vi "Move to Wavelength Inner (TRIAX).vi"(7 "Mono System # (0)":T1, 8 "error in (no error)":errorcluster, 10 "wavelength":dbl[unit], 11 "VISA resource name":refnum<visa-resource-name>) -> (0 "error out":errorcluster, 3 "VISA resource name out":refnum<visa-resource-name>)   [LabVIEW 2012, in "JY-SPEX-TRIAX.lvlib"]
doc: "Moves the spectrometer's grating to a specific wavelength according to the base grating (1200 grooves/mm).\n\n<B>Note: only works with TRIAX series monochromators.</B>"
uses:
  JY-SPEX-TRIAX.lvlib
  controls.llb/Monochromator System Number.ctl
  Spectrometer Config.vi
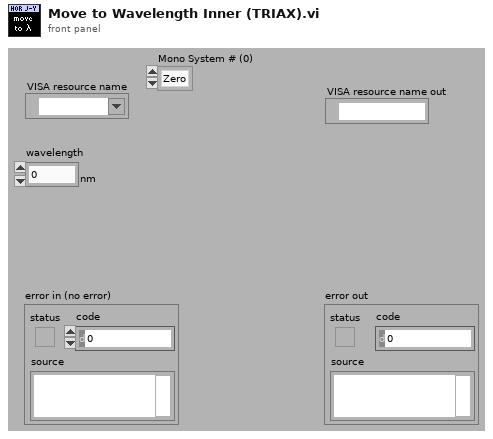
[diagram p1: front panel]
types:
  T1 = typedef "JY-SPEX-TRIAX.lvlib/Monochromator System Number.ctl" = enum16{"Zero", "One"}
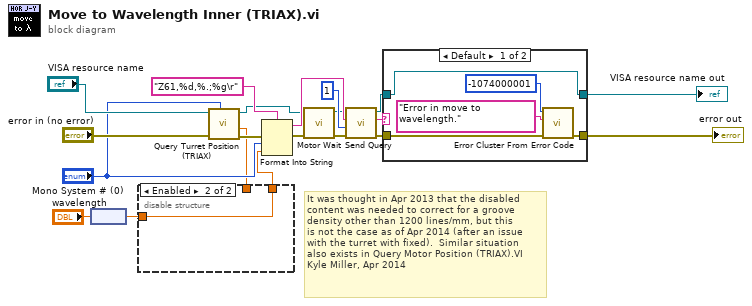
[diagram p0: block diagram]
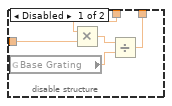
[diagram p2: hidden frame]
diagram:
  # "It was thought in Apr 2013 that the disabled\ncontent was needed to correct for a groove\ndensity other than 1200 lines/mm, but this\nis not the case as of Apr 2014 (after an issue\nwith the turret with fixed).  Similar situation\nalso exists in Query Motor Position (TRIAX).VI\nKyle Miller, Apr 2014"
  n1 = node("wavelength") -> (w3:dbl)
  n2 = call "Query Turret Position (TRIAX).vi"("Mono System # (0)"="Mono System # (0)", "error in (no error)"="error in (no error)", "VISA resource name"="VISA resource name") -> ("error out"=w7:errorcluster, "Groove Density"=w2:dbl[unit], "VISA resource name out"=w4:refnum<visa-resource-name>)  [unwired: 4 in, 2 out]
  n3 = disable-structure shown="Enabled" {
    disable-tunnel: w3 -> [w25 w26]
    disable-tunnel: w2 -> [w24 _]
    disable-tunnel: [w21 w26] -> w1
    frame Disabled {
      n4 = global read "Spectrometer Config.vi" "Base Grating"() -> (w22:dbl[unit])
      n5 = Multiply(x=w24, y=w25) -> (x*y=w23:dbl[unit])
      n6 = Divide(x=w23, y=w22) -> (x/y=w21:dbl)
    }
    frame Enabled {
    }
  }
  n7 = Format Into String(format string="Z61,%d,%.;%g\r", error in=w7, "Mono System # (0)", w1) -> (resulting string=w19:string, error out=w11:errorcluster)  [unwired: 1 in]
  n8 = call "Motor Wait.vi"("error in"=w11, "VISA resource name in"=w4) -> ("error out"=w10:errorcluster, "VISA resource name out"=w9:refnum<visa-resource-name>)  [unwired: 8 out]
  n9 = call "Send Query.vi"("error in (no error)"=w10, "byte count"=u32 1, "write buffer"=w19, "VISA resource name"=w9) -> ("error out"=w14:errorcluster, "read buffer"=w17:string, "VISA resource name out"=w16:refnum<visa-resource-name>)  [unwired: 5 out]
  n10 = case shown="Default" w17 {
    tunnel: w16 -> [w27 w33]
    tunnel: [w27 w33] -> w15
    tunnel: w14 -> [w29 w32]
    tunnel: [w28 w32] -> w13
    frame Default {
      n11 = call <vilib>:"Error Cluster From Error Code.vi"("error in (no error)"=w29, "error message (\"\")"="Error in move to wavelength." ("error message (\"\")"), "error code (0)"=-1074000001) -> ("error out"=w28:errorcluster)  [unwired: 1 in, 5 out]
    }
    frame "o" {
    }
  }
  "VISA resource name out" <- w15
  "error out" <- w13
